vi "Inline SubVIs.vi"(8 "error in (no error)":errorcluster, 10 "VIs to Inline":string[](array[string]), 11 "VI Reference In":refnum<vi>) -> (0 "error out":errorcluster, 3 "VI Reference Out":refnum<vi>)   [LabVIEW 2021]
panel:
  # "This VI takes a reference to the scripted VI and inlines sub VIs specified in the VIs to Inline input. \nInline = replace SubVI in the scripted block diagram with its contents"
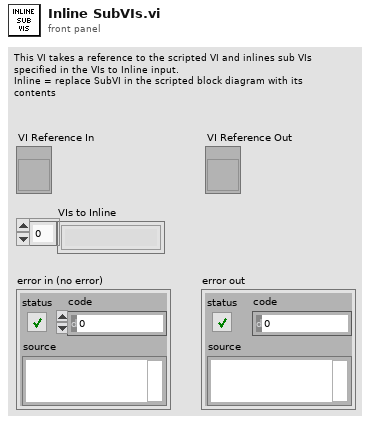
[diagram p1: front panel]
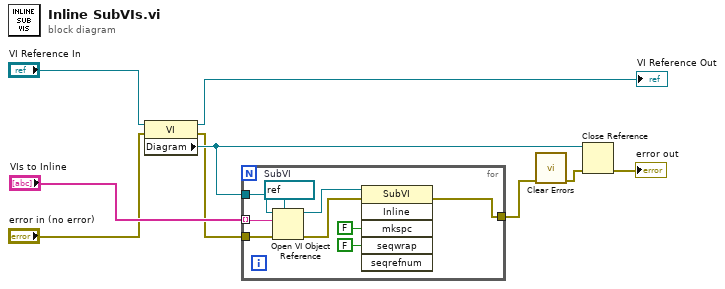
[diagram p0: block diagram]
diagram:
  n1 = property class="VI"(reference="VI Reference In", error in="error in (no error)") -> (reference out=→"VI Reference Out":refnum<vi>, error out=w1:errorcluster, "Diagram"=w4:refnum<vi>)
  n2 = for {
    tunnel: "VIs to Inline" -> [w18] mode=indexing
    tunnel: w4 -> [w17]
    tunnel: [w10] -> w6
    tunnel: w1 -> [w11]
    w16 = refnum<vi> refnum  # SubVI
    n3 = Open VI Object Reference(7:w16, 8:w11, 10:w18, 11:w17) -> (0:w15:errorcluster, 3:w14:refnum<vi>)
    n4 = invoke class="SubVI" method="Inline"(reference=w14, error in=w15, "mkspc"=FALSE ("Make Space in Block Diagram"), "seqwrap"=FALSE ("Wrap in Sequence")) -> (error out=w10:errorcluster)  [unwired: 2 in, 5 out]
  }
  n5 = call <vilib>:"Clear Errors.vi"("error in (no error)"=w6) -> ("error out"=w5:errorcluster)  [unwired: 5 in, 1 out]
  n6 = Close Reference(reference=w4, error in (no error)=w5) -> (error out=→"error out":errorcluster)
